vi "BDU绝缘电阻测试.vi"(8 "error in (no error)":errorcluster, 10 "等待时间（毫秒）":u32=10000, 11 "仪器实例 in":T1) -> (0 "错误输出":errorcluster, 2 "绝缘电阻":u16[](array[numeric]), 3 "仪器实例 out":T1)   [LabVIEW 2020]
uses:
  F:/F020/S7_1200 control/HslCommunication.dll
  S7_1200 control/HslCommunication.dll
  S7_1200 control/S7_1200 WriteBools.vi
  <instrlib>/Keithley 24XX/Keithley 24XX.lvlib
  S7_1200 control/S7_1200 control.lvlib
panel:
  # "F020绝缘电阻测试"
  # "仪器地址设置"
  # "kΩ"
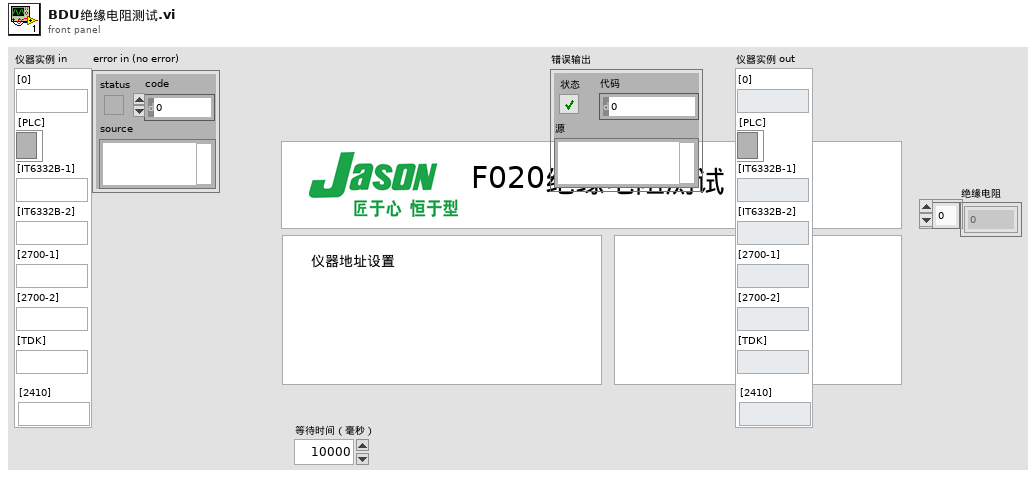
[diagram p1: front panel]
types:
  T1 = typedef "仪器实例.ctl" = cluster{"[0]":string, "[PLC]":refnum<k24>, "[IT6332B-1]":string, "[IT6332B-2]":string, "[2700-1]":string, "[2700-2]":string, "[TDK]":string, "[2410]":string}
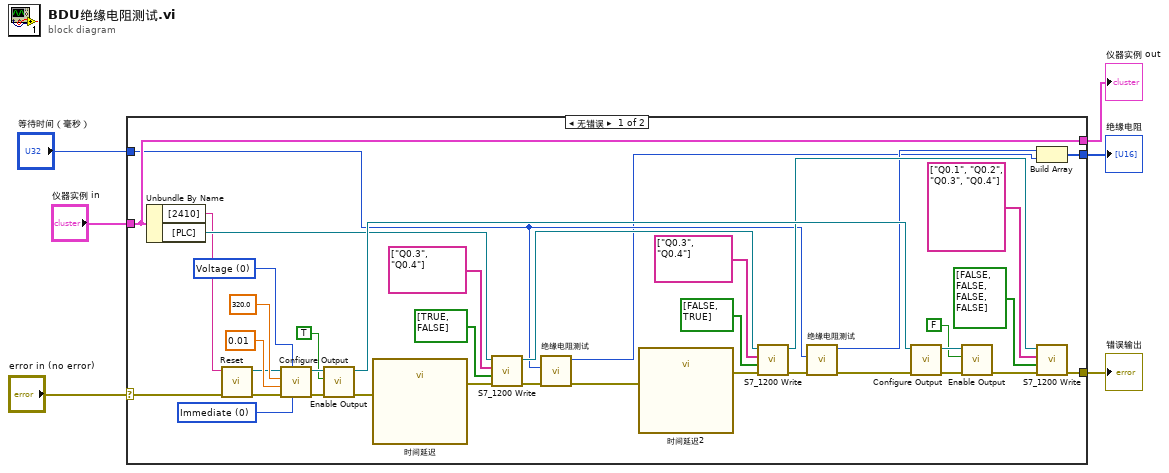
[diagram p0: block diagram]
diagram:
  n1 = case shown="无错误" "error in (no error)" {
    selector: "error in (no error)" -> [w12 w45]
    tunnel: "仪器实例 in" -> [w20 w46]
    tunnel: [w21 w45] -> w4
    tunnel: [w20 w46] -> w3
    tunnel: "等待时间（毫秒）" -> [w19 _]
    tunnel: [w16 _] -> w1
    frame No Error {
      w15 = u16 0 items=["Voltage", "Current"] ("Source Mode  (0: Voltage)")
      w43 = u16 0 items=["Immediate", "Triggered"] ("Output Type  (0: Immediate)")
      n2 = Unbundle By Name(w20) -> ("[2410]"=w13:string, "[PLC]"=w29:refnum<k24>)
      n3 = call <instrlib>:"Reset.vi"("error in (no error)"=w12, "VISA resource name"=w13) -> ("error out"=w11:errorcluster, "VISA resource name out"=w14:refnum<visa-resource-name>)  [unwired: 8 in]
      n4 = call <instrlib>:"Configure Output.vi"("Output Type  (0: Immediate)"=w43, "Source Mode  (0: Voltage)"=w15, "error in (no error)"=w11, "Compliance  Level (0.1)"=0.01, "Output Level (0)"=320.0, "VISA resource name"=w14) -> ("error out"=w42:errorcluster, "VISA resource name out"=w41:refnum<visa-resource-name>)  [unwired: 4 in]
      n5 = call <instrlib>:"Enable Output.vi"("error in (no error)"=w42, "Enable Output (T: Enable)"=TRUE, "VISA resource name"=w41) -> ("error out"=w10:errorcluster, "VISA resource name out"=w36:refnum<visa-resource-name>)  [unwired: 7 in]
      n6 = call "时间延迟"("error in (no error)"=w10) -> ("error out"=w9:errorcluster)  [unwired: 10 in]
      n7 = call-poly "S7_1200 Write.vi"("错误输入（无错误）"=w9, "values"=bool[] [TRUE, FALSE], "addresses"=string[] ["Q0.3", "Q0.4"], "引用"=w29) -> ("错误输出"=w27:errorcluster, "引用输出"=w28:refnum<k24>)  [unwired: 2 in]
      n8 = call "绝缘电阻测试.vi"("error in"=w27, "等待时间（毫秒）"=w19) -> ("error out"=w8:errorcluster, "绝缘电阻"=w17:u16)  [unwired: 8 in]
      n9 = call "时间延迟2"("error in (no error)"=w8) -> ("error out"=w7:errorcluster)  [unwired: 10 in]
      n10 = call-poly "S7_1200 Write.vi"("错误输入（无错误）"=w7, "values"=bool[] [FALSE, TRUE], "addresses"=string[] ["Q0.3", "Q0.4"], "引用"=w28) -> ("错误输出"=w26:errorcluster, "引用输出"=w24:refnum<k24>)  [unwired: 2 in]
      n11 = call "绝缘电阻测试.vi"("error in"=w26, "等待时间（毫秒）"=w19) -> ("error out"=w25:errorcluster, "绝缘电阻"=w18:u16)  [unwired: 8 in]
      n12 = call <instrlib>:"Configure Output.vi"("error in (no error)"=w25, "VISA resource name"=w36) -> ("error out"=w39:errorcluster, "VISA resource name out"=w38:refnum<visa-resource-name>)  [unwired: 8 in]
      n13 = call <instrlib>:"Enable Output.vi"("error in (no error)"=w39, "Enable Output (T: Enable)"=FALSE, "VISA resource name"=w38) -> ("error out"=w23:errorcluster)  [unwired: 7 in, 1 out]
      n14 = Build Array(w18, w17) -> (w16:u16[])
      n15 = call-poly "S7_1200 Write.vi"("错误输入（无错误）"=w23, "values"=bool[] [FALSE, FALSE, FALSE, FALSE], "addresses"=string[] ["Q0.1", "Q0.2", "Q0.3", "Q0.4"], "引用"=w24) -> ("错误输出"=w21:errorcluster)  [unwired: 2 in, 1 out]
    }
    frame Error {
    }
  }
  "错误输出" <- w4
  "仪器实例 out" <- w3
  "绝缘电阻" <- w1
